vi "Destroy.vi"(8 "error in (no error)":errorcluster, 11 "Writer (ARGB) in":refnum<class "Writer (ARGB).lvclass">) -> (0 "error out":errorcluster, 3 "Path":path)   [LabVIEW 2020, in "video_io.lvlib" / "Writer (ARGB).lvclass"]
uses:
  Writer (ARGB).lvclass
  Writer (ARGB).lvclass/Writer (ARGB).ctl
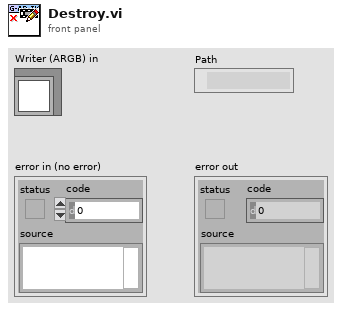
[diagram p1: front panel]
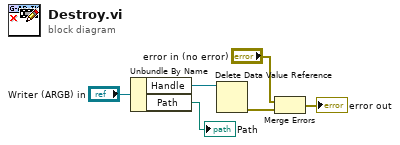
[diagram p0: block diagram]
diagram:
  n1 = Unbundle By Name("Writer (ARGB) in") -> ("Handle"=w4:refnum<data-value>, "Path"=→"Path":path)
  n2 = Delete Data Value Reference(data value reference=w4) -> (error out=w2:errorcluster)  [unwired: 1 in, 1 out]
  n3 = Merge Errors("error in (no error)", w2) -> (→"error out":errorcluster)
